vi "Set_Traverse_Position.vi"(3 "Simulate/Run":T3, 4 "Currently on Point":i32=11, 5 "Traverse line":T4 {"Row Duration (mins)" format="%#.1f"; "Row No" min=0; "Trace Gas Concentration (%)" min=0.0 format="%#.2f"; "Emission Rate (l/min)" format="%#.2f"; "Tunnel Speed" format="%#.2f"; "Start X" format="%#.2f"; "Start Y" format="%#.2f"; "Start Z" format="%#.2f"; "End X" format="%#.2f"; "End Y" format="%#.2f"; "End Z" format="%#.2f"; "Averaging time (min)" min=0.0 format="%#.2f"}) -> (0 "Status Cluster":T1)   [LabVIEW 2010]
uses:
  Traverse_cluster.ctl
  Spacing.ctl
  Controls/Multi_run_mode.ctl
  Controls/User_Specific_mode.ctl
  Status_Cluster.ctl
  Multi_Run_Status.ctl
  Trav_mode.ctl
  Globals/Trav_pos_global.vi
  Globals/Constants_global.vi
  Globals/Dynamic_call_global.ph.vi
panel:
  # "X           Y            Z"
  # "Start"
  # "End"
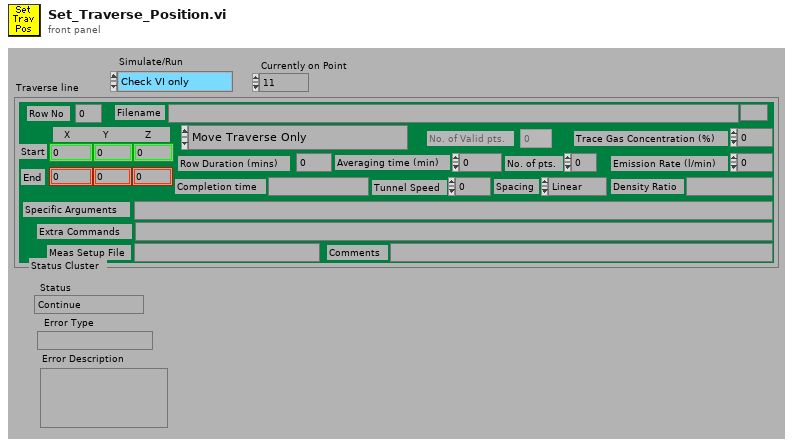
[diagram p1: front panel]
types:
  T1 = typedef "Status_Cluster.ctl" = cluster{"Status":T2, "Error Type":string, "Error Description":string}
  T2 = typedef "Multi_Run_Status.ctl" = enum16{"Continue", "Jump to Next Point", "Jump to Next Row", "Jump To Fall Back", "Terminate Run"}
  T3 = typedef "User_Specific_mode.ctl" = enum16{"Check VI only", "Run VI"}
  T4 = typedef "Traverse_cluster.ctl" = cluster{"Start X":dbl, "Start Y":dbl, "Start Z":dbl, "End X":dbl, "End Y":dbl, "End Z":dbl, "No. of pts.":i32, "Spacing":T5, "Filename":path, "Tunnel Speed":dbl, "Averaging time (min)":dbl, "Extra Commands":string, "Specific Arguments":string, "Emission Rate (l/min)":dbl, "Trace Gas Concentration (%)":dbl, "Density Ratio":string, "Comments":string, "Row No":i32, "Row Type Selector":T6, "Completion time":string, "Row Duration (mins)":dbl, "No. of Valid pts.":i32, "Meas Setup File":string}
  T5 = typedef "Spacing.ctl" = enum16{"Linear", "Log", "Gauss", "Specified", "N/A"}
  T6 = typedef "Multi_run_mode.ctl" = enum16{"Move Traverse Only", "Set Tunnel Speed Only", "Set Source Only", "Set Measurement Conditions", "Single Measurement", "Vertical Profile", "Lateral Profile", "Longitudinal Profile", "Explore Volume", "Multi-Axis Profile", "Auto Calibrate", "Meas Fast FID Bkgnd", "Check Beam Power", "Scanning Valve Measurement", "Run VI Named:", "Set ADAM Ch", "Wait (minutes)", "Send Message", "Synchronize With:", "Fall Back to this Row", "Turn Off Row Repeating", "Blank Row"}
  T7 = typedef "Trav_mode.ctl" = enum16{"Move traverse", "Read traverse position", "Teach Position"}
  T8 = cluster{"Name":string, "X":dbl, "Y":dbl, "Z":dbl}[]
  T9 = cluster{"Name":string, "X":dbl, "Y":dbl, "Z":dbl}
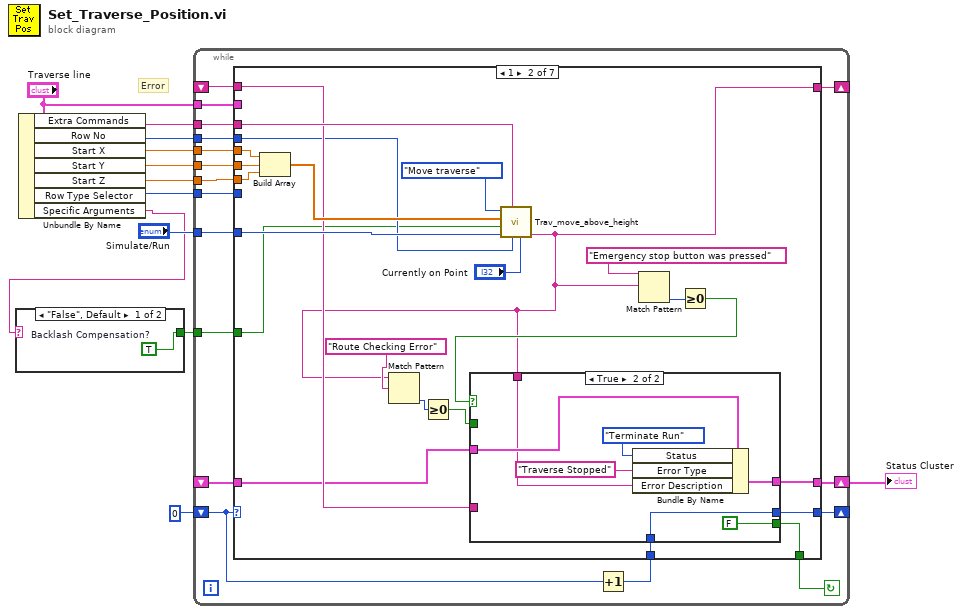
[diagram p0: block diagram]
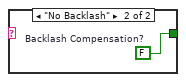
[diagram p2: hidden frame]
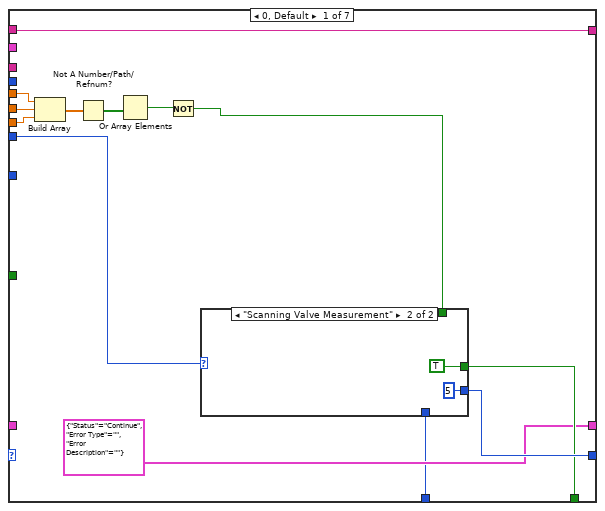
[diagram p3: hidden frame]
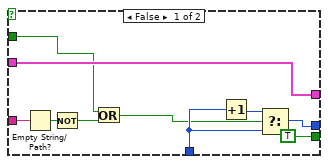
[diagram p5: hidden frame]
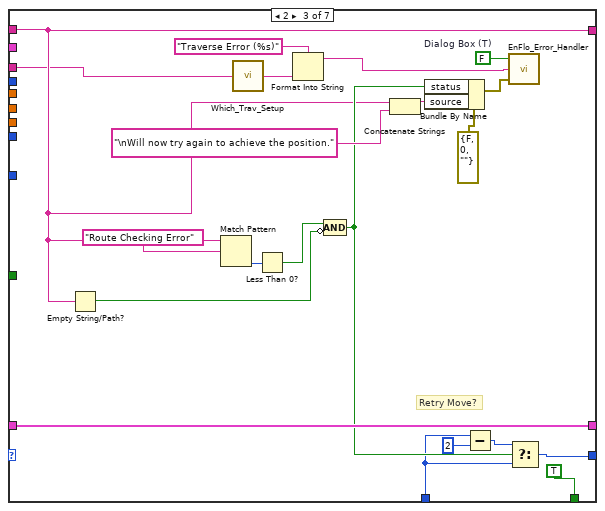
[diagram p6: hidden frame]
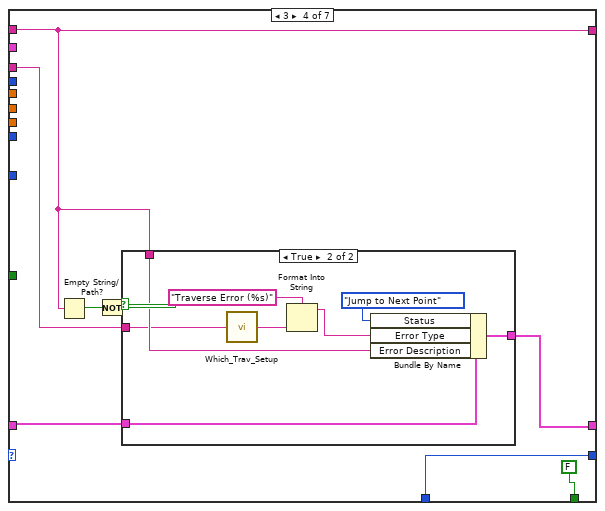
[diagram p7: hidden frame]
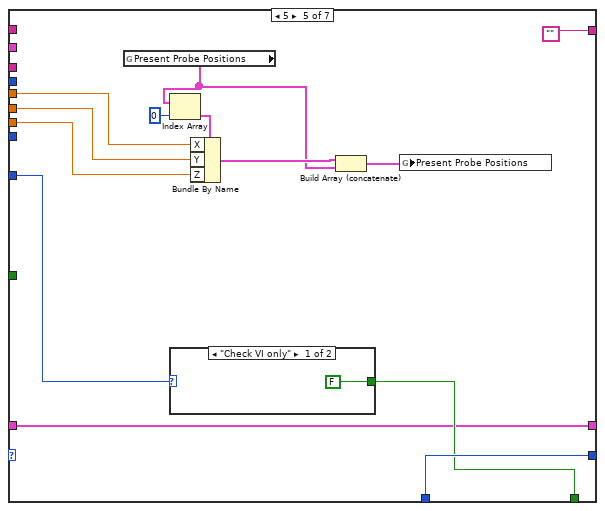
[diagram p9: hidden frame]
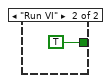
[diagram p10: hidden frame]
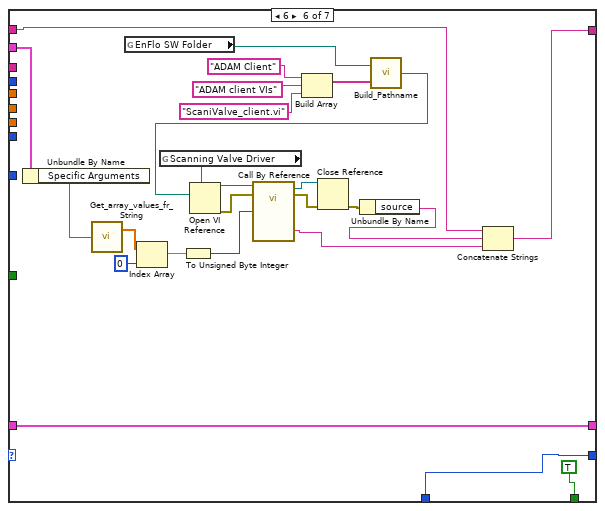
[diagram p11: hidden frame]
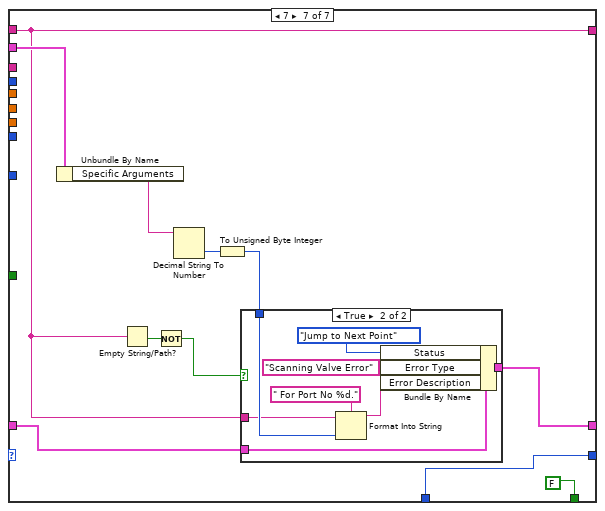
[diagram p12: hidden frame]
diagram:
  # "Error"
  n1 = Unbundle By Name("Traverse line") -> ("Extra Commands"=w11:string, "Row No"=w10:i32, "Start X"=w7:dbl, "Start Y"=w12:dbl, "Start Z"=w6:dbl, "Row Type Selector"=w8:T6, "Specific Arguments"=w2:string)
  n2 = case shown="\"False\", Default" w2 {
    tunnel: [w13 w14] -> w1
    frame "False", Default {
      w13 = TRUE  # Backlash Compensation?
    }
    frame "No Backlash" {
      w14 = FALSE  # Backlash Compensation?
    }
  }
  n3 = while {
    shift-left: _ -> [w16]
    shift-right: [w17] -> _
    shift-left: _ -> [w18]
    shift-right: [w19] -> w3
    tunnel: "Traverse line" -> [w20]
    tunnel: "Simulate/Run" -> [w21]
    tunnel: w6 -> [w22]
    tunnel: w12 -> [w23]
    tunnel: w7 -> [w24]
    tunnel: w8 -> [w29]
    shift-left: 0 -> [w27]
    shift-right: [w26] -> _
    tunnel: w10 -> [w30]
    tunnel: w11 -> [w31]
    tunnel: w1 -> [w15]
    stop <- w28 continue-if-true
    n4 = Increment(x=w27) -> (x+1=w25:i32)
    n5 = case shown="1" w27 {
      tunnel: w31 -> [_ w69 w92 w110 _ _ _]
      tunnel: w30 -> [_ w60 _ _ _ _ _]
      tunnel: w29 -> [w44 _ _ _ _ _ _]
      tunnel: [w42 w54 TRUE FALSE w132 TRUE FALSE] -> w28
      tunnel: [w43 w62 w95 w115 w134 w143 w167] -> w26
      tunnel: w25 -> [w40 w63 w96 w115 w134 w143 w167]
      tunnel: w24 -> [w36 w68 _ _ w137 _ _]
      tunnel: w23 -> [w37 w67 _ _ w136 _ _]
      tunnel: w22 -> [w38 w66 _ _ w135 _ _]
      tunnel: w21 -> [_ w64 _ _ w133 _ _]
      tunnel: w20 -> [_ _ _ _ _ w160 w176]
      tunnel: [T1 {"Status"=enum."Continue", "Error Type"="", "Error Description"=""} ("Status Cluster") w56 w104 w116 w131 w151 w173] -> w19
      tunnel: w18 -> [_ w55 w104 w117 w131 w151 w174]
      tunnel: [w39 w52 w94 w112 "" w144 w168] -> w17
      tunnel: w16 -> [w39 w61 w94 w112 _ w142 w168]
      tunnel: w15 -> [_ w49 _ _ _ _ _]
      frame 0, Default {
        n6 = Build Array(w36, w37, w38) -> (w35:dbl[])
        n7 = Not A Number/Path/Refnum?(number/path/refnum=w35) -> (NaN/Path/Refnum?=w34:bool[])
        n8 = Or Array Elements(Boolean array=w34) -> (logical OR=w33:bool)
        n9 = Not(x=w33) -> (.not. x?=w32:bool)
        n10 = case shown="\"Scanning Valve Measurement\"" w44 {
          tunnel: [w45 5] -> w43
          tunnel: [w46 TRUE] -> w42
          tunnel: w32 -> [w46 _]
          tunnel: w40 -> [w45 _]
          frame "Move Traverse Only", Default {
          }
          frame "Scanning Valve Measurement" {
          }
        }
      }
      frame 1 {
        n11 = Build Array(w68, w67, w66) -> (w65:dbl[])
        n12 = call "Trav_move_above_height.vi"("Currently on Point"="Currently on Point", "Row Number"=w60, "Extra Command String"=w69, "Simulate/Run"=w64, "Backlash Compensation?"=w49, "New Position"=w65, "Mode"=Trav_mode."Move traverse") -> ("Error String"=w52:string)  [unwired: 1 in, 3 out]
        n13 = Match Pattern(string=w52, regular expression="Route Checking Error") -> (offset past match=w51:i32)  [unwired: 4 out]
        n14 = Greater Or Equal To 0?(x=w51) -> (x >= 0?=w50:bool)
        n15 = Match Pattern(string=w52, regular expression="Emergency stop button was pressed") -> (offset past match=w58:i32)  [unwired: 4 out]
        n16 = Greater Or Equal To 0?(x=w58) -> (x >= 0?=w57:bool)
        n17 = case shown="True" w57 {
          tunnel: w63 -> [w80 w83]
          tunnel: [w79 w83] -> w62
          tunnel: w61 -> [w77 _]
          tunnel: [w76 w85] -> w56
          tunnel: w55 -> [w76 w86]
          tunnel: w52 -> [_ w84]
          tunnel: [TRUE FALSE] -> w54
          tunnel: w50 -> [w73 _]
          frame False {
            n18 = Empty String/Path?(string/path=w77) -> (empty?=w78:bool)
            n19 = Not(x=w78) -> (.not. x?=w74:bool)
            n20 = Or(x=w73, y=w74) -> (x .or. y?=w72:bool)
            n21 = Increment(x=w80) -> (x+1=w81:i32)
            n22 = Select(t=w81, s=w72, f=w80) -> (s? t:f=w79:i32)
          }
          frame True {
            n23 = Bundle By Name(cluster=w86, "Status"=Multi_Run_Status."Terminate Run", "Error Type"="Traverse Stopped" ("t"), "Error Description"=w84) -> (w85:T1)
          }
        }
      }
      frame 2 {
        w107 = FALSE  # Dialog Box (T)
        # "Retry Move?"
        n24 = Empty String/Path?(string/path=w94) -> (empty?=w93:bool)
        n25 = Match Pattern(string=w94, regular expression="Route Checking Error" ("String to match")) -> (offset past match=w101:i32)  [unwired: 4 out]
        n26 = call "Which_Trav_Setup.vi"("Extra Command String"=w92) -> ("Traverse Setup"=w90:string)
        n27 = Less Than 0?(x=w101) -> (x < 0?=w100:bool)
        n28 = Format Into String(format string="Traverse Error (%s)" ("t"), w90) -> (resulting string=w89:string)  [unwired: 2 in, 1 out]
        n29 = Compound Arithmetic op=AND(w100, invert w93) -> (w99:bool)
        n30 = Concatenate Strings(w94, "\nWill now try again to achieve the position." ("Substring")) -> (w106:string)
        n31 = Bundle By Name(cluster=errorcluster {"status"=FALSE, "code"=0, "source"=""} ("error in (no error)"), "status"=w99, "source"=w106) -> (w108:errorcluster)
        n32 = Subtract(x=w96, y=2) -> (x-y=w97:i32)
        n33 = call "EnFlo_Error_Handler.vi"("error in (no error)"=w108, "Error Type"=w89, "Dialog Box (T)"=w107) -> ()  [unwired: 3 out]
        n34 = Select(t=w97, s=w99, f=w96) -> (s? t:f=w95:i32)
      }
      frame 3 {
        n35 = Empty String/Path?(string/path=w112) -> (empty?=w113:bool)
        n36 = Not(x=w113) -> (.not. x?=w111:bool)
        n37 = case shown="True" w111 {
          tunnel: w117 -> [w118 w126]
          tunnel: [w118 w124] -> w116
          tunnel: w112 -> [_ w123]
          tunnel: w110 -> [_ w119]
          frame False {
          }
          frame True {
            n38 = call "Which_Trav_Setup.vi"("Extra Command String"=w119) -> ("Traverse Setup"=w121:string)
            n39 = Format Into String(format string="Traverse Error (%s)" ("t"), w121) -> (resulting string=w120:string)  [unwired: 2 in, 1 out]
            n40 = Bundle By Name(cluster=w126, "Status"=Multi_Run_Status."Jump to Next Point", "Error Type"=w120, "Error Description"=w123) -> (w124:T1)
          }
        }
      }
      frame 5 {
        n41 = global read "Trav_pos_global.vi" "Present Probe Positions"() -> (w128:T8)
        n42 = Index Array(array=w128, index=0 ("Index")) -> (element=w139:T9)
        n43 = case shown="\"Check VI only\"" w133 {
          tunnel: [FALSE TRUE] -> w132
          frame "Check VI only" {
          }
          frame "Run VI" {
          }
        }
        n44 = Bundle By Name(cluster=w139, "X"=w137, "Y"=w136, "Z"=w135) -> (w129:T9)
        n45 = Build Array (concatenate)(w129, w128) -> (w127:T8)
        n46 = global write "Trav_pos_global.vi" "Present Probe Positions"(w127) -> ()
      }
      frame 6 {
        n47 = Unbundle By Name(w160) -> ("Specific Arguments"=w148:string)
        n48 = call "Get_array_values_fr_String.vi"("String Value"=w148) -> ("Numeric Array"=w150:dbl[])  [unwired: 1 out]
        n49 = global read "Constants_global.vi" "EnFlo SW Folder"() -> (w154:path)
        n50 = Index Array(array=w150, index=0) -> (element=w147:dbl)
        n51 = global read "Dynamic_call_global.ph.vi" "Scanning Valve Driver"() -> (w161:refnum<vi>)
        n52 = To Unsigned Byte Integer(number=w147) -> (unsigned 8bit integer=w159:u8)
        n53 = Build Array("ADAM Client", "ADAM client VIs", "ScaniValve_client.vi") -> (w155:string[])
        n54 = call "Build_Pathname.vi"("Output Array"=w155, "Pathname"=w154) -> ("Appended path"=w153:path)
        n55 = Open VI Reference(type specifier VI Refnum (for type only)=w161, vi path=w153) -> (vi reference=w162:refnum<vi>, error out=w163:errorcluster)  [unwired: 2 in, 2 out]
        n56 = call-by-ref "?"(reference=w162, error in=w163, "Port Number"=w159) -> (reference out=w165:refnum<vi>, error out=w164:errorcluster, "Error String"=w145:string)  [unwired: 2 out]
        n57 = Close Reference(reference=w165, error in (no error)=w164) -> (error out=w166:errorcluster)
        n58 = Unbundle By Name(w166) -> ("source"=w146:string)
        n59 = Concatenate Strings(w142, w146, w145) -> (w144:string)
      }
      frame 7 {
        n60 = Unbundle By Name(w176) -> ("Specific Arguments"=w177:string)
        n61 = Empty String/Path?(string/path=w168) -> (empty?=w170:bool)
        n62 = Not(x=w170) -> (.not. x?=w169:bool)
        n63 = Decimal String To Number(string=w177) -> (number=w175:i32)  [unwired: 3 out]
        n64 = To Unsigned Byte Integer(number=w175) -> (unsigned 8bit integer=w172:u8)
        n65 = case shown="True" w169 {
          tunnel: w174 -> [w178 w186]
          tunnel: [w178 w183] -> w173
          tunnel: w172 -> [_ w181]
          tunnel: w168 -> [_ w179]
          frame False {
          }
          frame True {
            n66 = Format Into String(format string=" For Port No %d." ("Format String"), initial string=w179, w181) -> (resulting string=w180:string)  [unwired: 1 in, 1 out]
            n67 = Bundle By Name(cluster=w186, "Status"=Multi_Run_Status."Jump to Next Point", "Error Type"="Scanning Valve Error" ("t"), "Error Description"=w180) -> (w183:T1)
          }
        }
      }
    }
  }
  "Status Cluster" <- w3
